vi "InitializeRings.vi"(8 "error in (no error)":errorcluster, 11 "Maui Manager in":refnum<class "Maui Manager.lvclass">) -> (0 "error out":errorcluster, 3 "Maui Manager out":refnum<class "Maui Manager.lvclass">)   [LabVIEW 2019, in "Maui Manager.lvclass"]
uses:
  Maui Manager.lvclass
  e917bdc8-0184-432d-91b1-c96dcc8050f0.vi
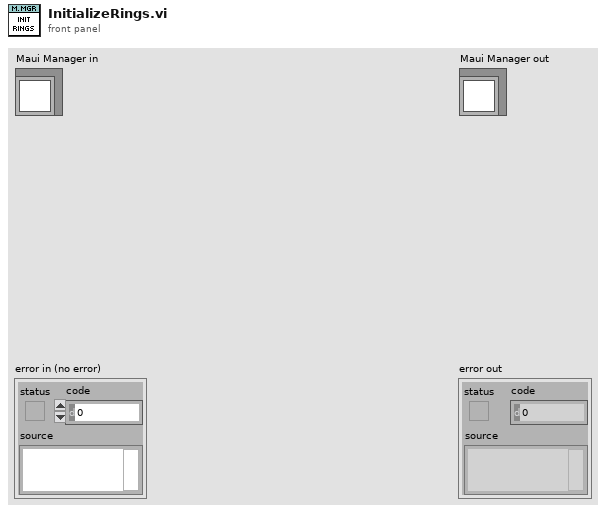
[diagram p1: front panel]
types:
  T1 = cluster{"Control":refnum<vi>, "Subpanel":refnum<vi>, "Active":i32, "Ctrl Class":string}[]
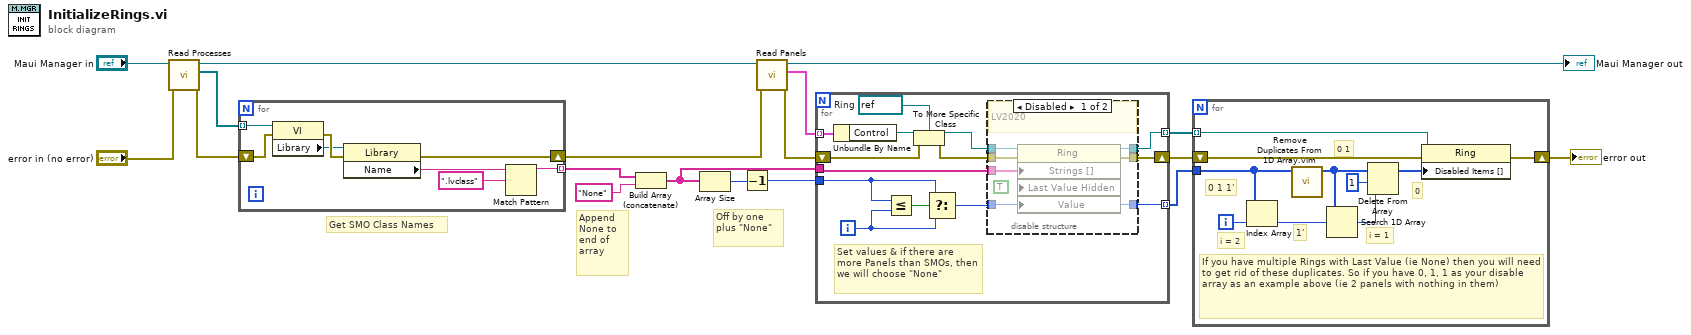
[diagram p0: block diagram]
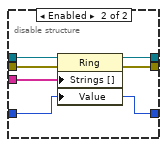
[diagram p2: hidden frame]
diagram:
  # "Off by one plus \"None\""
  # "Append None to end of array"
  # "Get SMO Class Names"
  n1 = call "Read Processes.vi"("error in (no error)"="error in (no error)", "Maui Manager in"="Maui Manager in") -> ("error out"=w17:errorcluster, "Processes"=w11:refnum<vi>[], "Maui Manager out"=w9:refnum<class "Maui Manager.lvclass">)  [unwired: 7 in]
  n2 = for {
    tunnel: [w20] -> w6 mode=indexing
    tunnel: w11 -> [w19] mode=indexing
    shift-right: [w26] -> w16
    shift-left: w17 -> [w25]
    n3 = property class="VI"(reference=w19, error in=w25) -> (error out=w24:errorcluster, "Library"=w22:refnum<vi>)  [unwired: 1 out]
    n4 = property class="Library"(reference=w22, error in=w24) -> (error out=w26:errorcluster, "Name"=w21:string)  [unwired: 1 out]
    n5 = Match Pattern(string=w21, regular expression=".lvclass") -> (before substring=w20:string)  [unwired: 1 in, 3 out]
  }
  n6 = Build Array (concatenate)(w6, "None") -> (w7:string[])
  n7 = Array Size(array=w7) -> (size(s)=w3:i32)
  n8 = Decrement(x=w3) -> (x-1=w1:i32)
  n9 = call "Read Panels.vi"("error in (no error)"=w16, "Maui Manager in"=w9) -> ("error out"=w15:errorcluster, "Panels"=w5:T1, "Maui Manager out"=→"Maui Manager out":refnum<class "Maui Manager.lvclass">)  [unwired: 7 in]
  n10 = for {
    tunnel: w5 -> [w34] mode=indexing
    tunnel: w7 -> [w35]
    tunnel: w1 -> [w33]
    tunnel: [w27] -> w2 mode=indexing
    tunnel: [w29] -> w4 mode=indexing
    shift-right: [w40] -> w14
    shift-left: w15 -> [w39]
    i -> [w31]
    w36 = refnum<vi> refnum  # Ring
    # "Set values & if there are more Panels than SMOs, then we will choose \"None\""
    n11 = Unbundle By Name(w34) -> ("Control"=w37:refnum<vi>)
    n12 = Less Or Equal?(x=w33, y=w31) -> (x <= y?=w32:bool)
    n13 = To More Specific Class(target class=w36, reference=w37, error in=w39) -> (specific class reference=w30:refnum<vi>, error out=w38:errorcluster)
    n14 = Select(t=w33, s=w32, f=w31) -> (s? t:f=w28:i32)
    n15 = disable-structure shown="Disabled" {
      disable-tunnel: [w46 w52] -> w40
      disable-tunnel: w38 -> [w45 w51]
      disable-tunnel: w35 -> [w44 w50]
      disable-tunnel: w30 -> [w43 w49]
      disable-tunnel: [w42 w48] -> w29
      disable-tunnel: w28 -> [w41 w47]
      disable-tunnel: [w41 w47] -> w27
      frame Disabled {
        (unwired) TRUE ("Last Value Hidden")
        # "LV2020"
        n16 = property class="Ring" props=["Strings []", "Last Value Hidden", "Value"](reference=w43, error in=w45, "Strings []"=w44, "Value"=w41) -> (reference out=w42:refnum<vi>, error out=w46:errorcluster)  [unwired: 1 in]
      }
      frame Enabled {
        n17 = property class="Ring"(reference=w49, error in=w51, "Strings []"=w50, "Value"=w47) -> (reference out=w48:refnum<vi>, error out=w52:errorcluster)
      }
    }
  }
  n18 = for {
    tunnel: w4 -> [w60] mode=indexing
    tunnel: w2 -> [w53]
    shift-right: [w61] -> w13
    shift-left: w14 -> [w62]
    i -> [w58]
    # "0"
    # "i = 1"
    # "0 1"
    # "1'"
    # "i = 2"
    # "0 1 1'"
    # "If you have multiple Rings with Last Value (ie None) then you will need to get rid of these duplicates. So if you have 0, 1, 1 as your disable array as an example above (ie 2 panels with nothing in them)"
    n19 = Index Array(array=w53, index=w58) -> (element=w57:i32)
    n20 = call "Remove Duplicates From 1D Array.vim"("array"=w53) -> ("array with duplicates removed"=w54:i32[])  [unwired: 10 in]
    n21 = Search 1D Array(1D array=w54, element=w57) -> (index of element=w56:i32)  [unwired: 1 in]
    n22 = Delete From Array(array=w54, length=1, index=w56) -> (array with subset deleted=w55:i32[])  [unwired: 1 out]
    n23 = property class="Ring"(reference=w60, error in=w62, "Disabled Items []"=w55) -> (error out=w61:errorcluster)  [unwired: 1 out]
  }
  "error out" <- w13
